vi "Save Window Position.vi"(8 "error in":errorcluster, 11 "VI Refnum":refnum<vi>) -> (0 "error out":errorcluster)   [LabVIEW 2020, in "Peek Window.lvlib"]
uses:
  Peek Window.lvlib
  <resource>/dialog/lvconfig.llb/LV Config Write String.vi
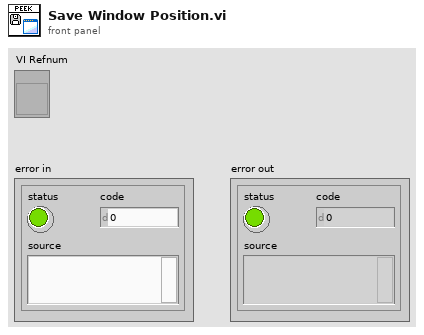
[diagram p1: front panel]
types:
  T1 = typedef "LVRectTypeDef.ctl" = cluster{"Left":i16, "Top":i16, "Right":i16, "Bottom":i16}
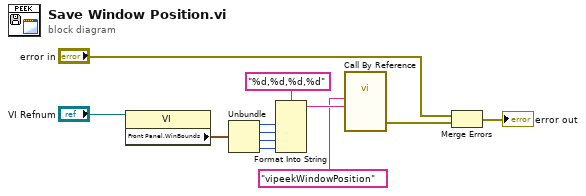
[diagram p0: block diagram]
diagram:
  n1 = property class="VI"(reference="VI Refnum") -> ("Front Panel.WinBounds"=w3:T1)  [unwired: 1 in, 2 out]
  n2 = Unbundle(w3) -> ("Left"=w9:i16, "Top"=w8:i16, "Right"=w7:i16, "Bottom"=w6:i16)
  n3 = Format Into String(format string="%d,%d,%d,%d", w9, w8, w7, w6) -> (resulting string=w4:string)  [unwired: 2 in, 1 out]
  n4 = call-by-ref "?"("value"=w4, "key"="vipeekWindowPosition" ("Name")) -> ("error out"=w2:errorcluster)  [unwired: 3 in, 6 out]
  n5 = Merge Errors("error in", w2) -> (→"error out":errorcluster)
